vi "PrefDlgRequest.vi"(8 "error in (no error)":errorcluster, 10 "Module Name":string, 11 "Module ID":i32) -> (0 "error out":errorcluster)   [LabVIEW 2018, in "Test.lvclass"]
uses:
  Test.lvclass
  <vilib>/Utility/error.llb/Error Cluster From Error Code.vi
  <vilib>/ErrorRing/Error Ring.xnode
  Sync/SyncPlugins/SyncPluginBase/SyncPluginBase.lvclass
  FGen/FgenPlugins/FgenPluginBaseClass/FgenPluginsBase.lvclass
  Scope/ScopeModule/ScopeModule.lvlib
  Digitizer/DigitizerPlugins/DigitizerBaseClass/DigitizerBase.lvclass
  Sensor/SensorModule/SensorModule.lvlib
  Analysis/AnalysisPlugins/AnalysisPluginBaseClass/AnalysisPluginsBase.lvclass
  AcPwr/AcPwrModule/AcPwrModule.lvlib
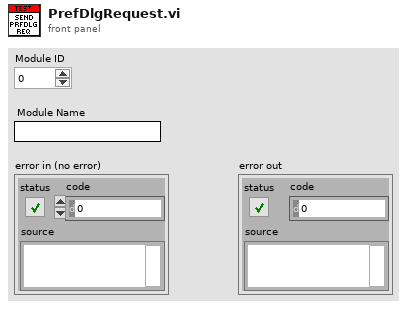
[diagram p1: front panel]
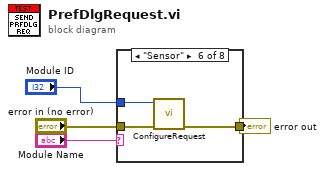
[diagram p0: block diagram]
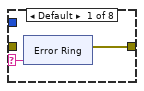
[diagram p2: hidden frame]
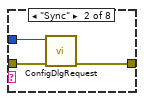
[diagram p3: hidden frame]
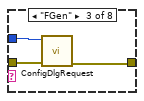
[diagram p4: hidden frame]
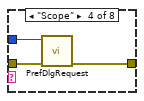
[diagram p5: hidden frame]
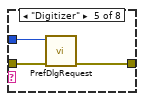
[diagram p6: hidden frame]
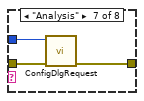
[diagram p7: hidden frame]
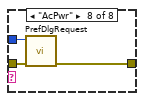
[diagram p8: hidden frame]
diagram:
  n1 = case shown="\"Sensor\"" "Module Name" {
    selector: "Module Name" -> [w6 _ _ _ _ _ _ _]
    tunnel: "Module ID" -> [_ w16 w19 w20 w25 w28 w31 w32]
    tunnel: "error in (no error)" -> [_ w15 w18 w22 w24 w27 w30 w33]
    tunnel: [w5 w14 w17 w21 w23 w26 w29 w34] -> w2
    frame Default {
      n2 = xnode "Error Ring"("parameter 0"=w6) -> ("error out"=w5:errorcluster)
    }
    frame "Sync" {
      n3 = call "ConfigDlgRequest.vi"("error in (no error)"=w15, "ModuleID"=w16) -> ("error out"=w14:errorcluster)  [unwired: 9 in]
    }
    frame "FGen" {
      n4 = call "ConfigDlgRequest.vi"("error in (no error)"=w18, "ModuleID"=w19) -> ("error out"=w17:errorcluster)  [unwired: 9 in]
    }
    frame "Scope" {
      n5 = call "PrefDlgRequest.vi"("error in (no error)"=w22, "ModuleID"=w20) -> ("error out"=w21:errorcluster)  [unwired: 9 in]
    }
    frame "Digitizer" {
      n6 = call "PrefDlgRequest.vi"("error in (no error)"=w24, "ModuleID"=w25) -> ("error out"=w23:errorcluster)  [unwired: 9 in]
    }
    frame "Sensor" {
      n7 = call "ConfigureRequest.vi"("error in (no error)"=w27, "ModuleID"=w28) -> ("error out"=w26:errorcluster)  [unwired: 9 in]
    }
    frame "Analysis" {
      n8 = call "ConfigDlgRequest.vi"("error in (no error)"=w30, "ModuleID"=w31) -> ("error out"=w29:errorcluster)  [unwired: 9 in]
    }
    frame "AcPwr" {
      n9 = call "PrefDlgRequest.vi"("error in (no error)"=w33, "ModuleID"=w32) -> ("error out"=w34:errorcluster)  [unwired: 9 in]
    }
  }
  "error out" <- w2
